vi "Read channel type.vi"(8 "error in (no error)":errorcluster, 11 "Channel group in":refnum<class "Channel group.lvclass">) -> (0 "error out":errorcluster, 2 "channel type":string, 3 "Channel group out":refnum<class "Channel group.lvclass">)   [LabVIEW 2016, in "FPGA RM Shared API.lvlib" / "Channel group.lvclass"]
uses:
  Channel group.lvclass
  Channel group.lvclass/Channel group.ctl
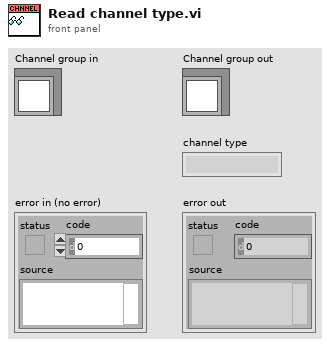
[diagram p1: front panel]
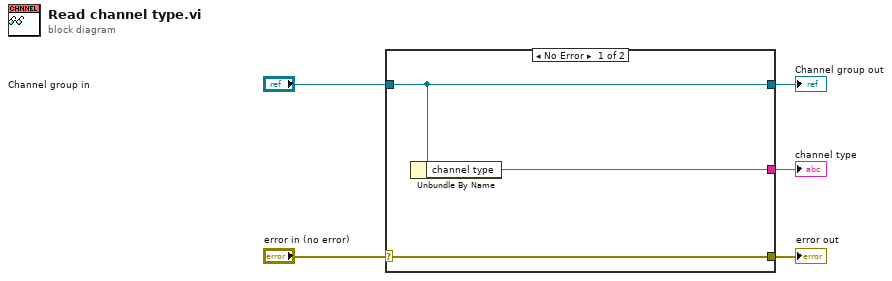
[diagram p0: block diagram]
diagram:
  n1 = case shown="No Error" "error in (no error)" {
    selector: "error in (no error)" -> [w8 w9]
    tunnel: [w8 w9] -> w4
    tunnel: [w7 w10] -> w2
    tunnel: "Channel group in" -> [w7 w10]
    tunnel: [w6 _] -> w1
    frame No Error {
      n2 = Unbundle By Name(w7) -> ("channel type"=w6:string)
    }
    frame Error {
    }
  }
  "error out" <- w4
  "Channel group out" <- w2
  "channel type" <- w1
